vi "Close vi references.vi"(8 "error in":errorcluster, 11 "Data Cluster":T1) -> (0 "error out":errorcluster)   [LabVIEW 2021, in "Panther Dashboard.lvlib"]
uses:
  Panther Dashboard.lvlib
  Module Data--cluster.ctl
  Maps List and refs--cluster.ctl
  <vilib>/National Instruments/Tree Map/Tree Map Data.ctl
  DQMH Modules Info--cluster.ctl
  Module type--enum.ctl
  Project References--cluster.ctl
  <vilib>/National Instruments/Tree Map/Tree Map.lvlib
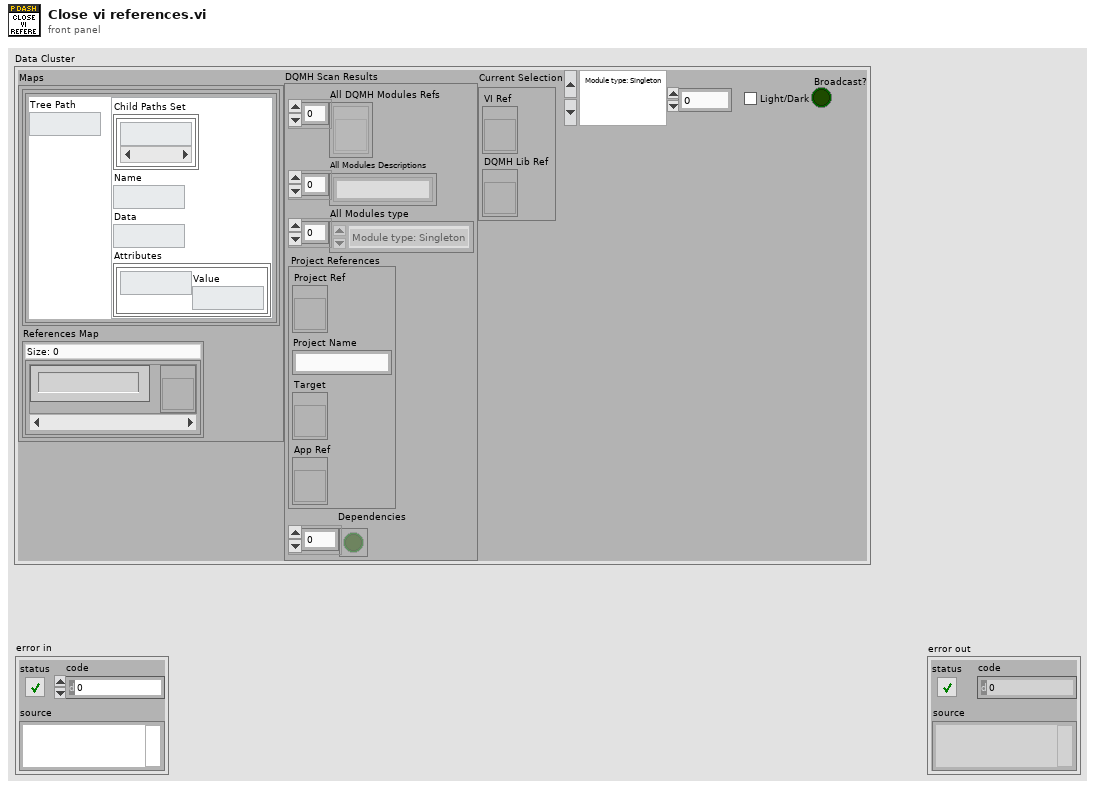
[diagram p1: front panel]
types:
  T1 = typedef "Panther Dashboard.lvlib/Module Data--cluster.ctl" = cluster{"Maps":T2, "DQMH Scan Results":T4, "Current Selection":cluster{"VI Ref":refnum<vi>, "DQMH Lib Ref":refnum<vi>}, "Module type":T5, "Module ID":i32, "Theme":bool, "Broadcast?":bool}
  T2 = typedef "Panther Dashboard.lvlib/Maps List and refs--cluster.ctl" = cluster{"Tree Map":T3, "References Map":map{string, refnum<vi>}}
  T3 = typedef "Tree Map.lvlib/Tree Map Data.ctl" = map{string, cluster{"Child Paths Set":set{string}, "Name":string, "Data":string, "Attributes":map{string, string}}}
  T4 = typedef "Panther Dashboard.lvlib/DQMH Modules Info--cluster.ctl" = cluster{"All DQMH Modules Refs":refnum<vi>[], "All Modules Descriptions":string[], "All Modules type":T5[], "Project References":T6, "Dependencies":bool[]}
  T5 = typedef "Panther Dashboard.lvlib/Module type--enum.ctl" = enum16{"Module type: Singleton", "Module type: Cloneable"}
  T6 = typedef "Panther Dashboard.lvlib/Project References--cluster.ctl" = cluster{"Project Ref":refnum<vi>, "Project Name":string, "Target":refnum<vi>, "App Ref":refnum<vi>}
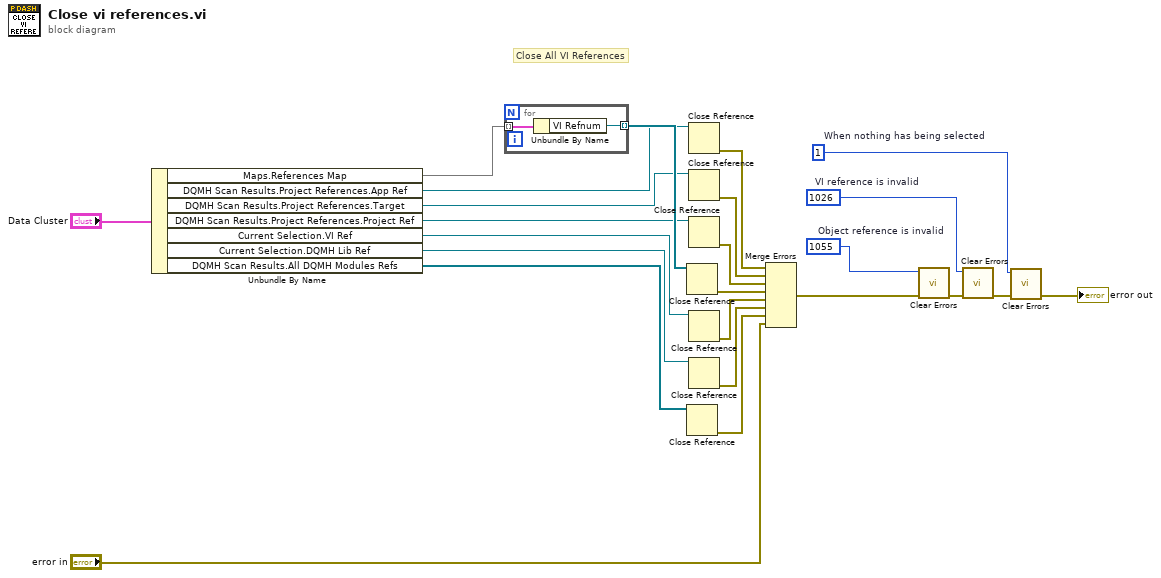
[diagram p0: block diagram]
diagram:
  w1 = 1  # When nothing has being selected
  w6 = 1026  # VI reference is invalid
  w7 = 1055  # Object reference is invalid
  # "Close All VI References"
  n1 = Unbundle By Name("Data Cluster") -> ("Maps.References Map"=w2:map{string, refnum<vi>}, "DQMH Scan Results.Project References.App Ref"=w5:refnum<vi>, "DQMH Scan Results.Project References.Target"=w4:refnum<vi>, "DQMH Scan Results.Project References.Project Ref"=w3:refnum<vi>, "Current Selection.VI Ref"=w10:refnum<vi>, "Current Selection.DQMH Lib Ref"=w9:refnum<vi>, "DQMH Scan Results.All DQMH Modules Refs"=w8:refnum<vi>[])
  n2 = for {
    tunnel: [w26] -> w12 mode=indexing
    tunnel: w2 -> [w25] mode=indexing
    n3 = Unbundle By Name(w25) -> ("VI Refnum"=w26:refnum<vi>)
  }
  n4 = Close Reference(reference=w12) -> (error out=w24:errorcluster)  [unwired: 1 in]
  n5 = Close Reference(reference=w8) -> (error out=w21:errorcluster)  [unwired: 1 in]
  n6 = Close Reference(reference=w5) -> (error out=w18:errorcluster)  [unwired: 1 in]
  n7 = Close Reference(reference=w4) -> (error out=w17:errorcluster)  [unwired: 1 in]
  n8 = Close Reference(reference=w3) -> (error out=w16:errorcluster)  [unwired: 1 in]
  n9 = Close Reference(reference=w10) -> (error out=w23:errorcluster)  [unwired: 1 in]
  n10 = Close Reference(reference=w9) -> (error out=w22:errorcluster)  [unwired: 1 in]
  n11 = Merge Errors(w18, w17, w16, w24, w23, w22, w21, "error in") -> (w20:errorcluster)
  n12 = call <vilib>:"Clear Errors.vi"("error in (no error)"=w20, "specific error code to clear (0: all)"=w7) -> ("error out"=w19:errorcluster)  [unwired: 4 in, 1 out]
  n13 = call <vilib>:"Clear Errors.vi"("error in (no error)"=w19, "specific error code to clear (0: all)"=w6) -> ("error out"=w15:errorcluster)  [unwired: 4 in, 1 out]
  n14 = call <vilib>:"Clear Errors.vi"("error in (no error)"=w15, "specific error code to clear (0: all)"=w1) -> ("error out"=→"error out":errorcluster)  [unwired: 4 in, 1 out]
